vi "oa_TV Ptbypt Interpolation (NChan).vi"(5 "reset? (F)":bool, 6 "buffer size":i32[](array[numeric]), 8 "error in (no error)":errorcluster, 9 "dX":dbl[](array[numeric]), 10 "Y":cluster{dbl[]}[](array[cluster]), 11 "X":cluster{dbl[]}[](array[cluster])) -> (0 "error out":errorcluster, 1 "X0":dbl[](array[numeric]), 2 "resampled X":cluster{dbl[]}[](array[cluster]), 3 "resampled Y":cluster{dbl[]}[](array[cluster]))   [LabVIEW 2017, in "SoundVib_Torsional.lvlib"]
uses:
  <vilib>/addons/Sound and Vibration/Order Analysis/Torsional Vibration/SoundVib_Torsional.lvlib
  <vilib>/Analysis/1siggen.llb/Ramp Pattern by Samples.vi
  <vilib>/gmath/NI_Gmath.lvlib
  <vilib>/Analysis/NI_AALBase.lvlib
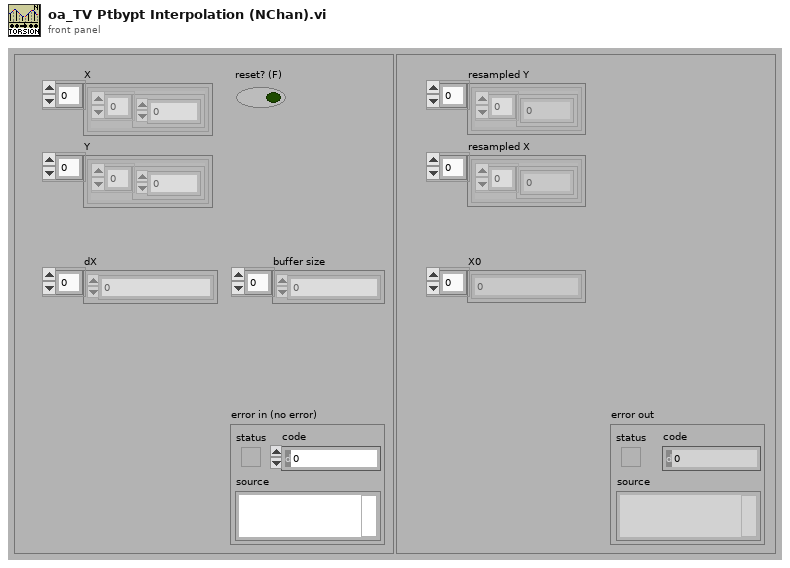
[diagram p1: front panel]
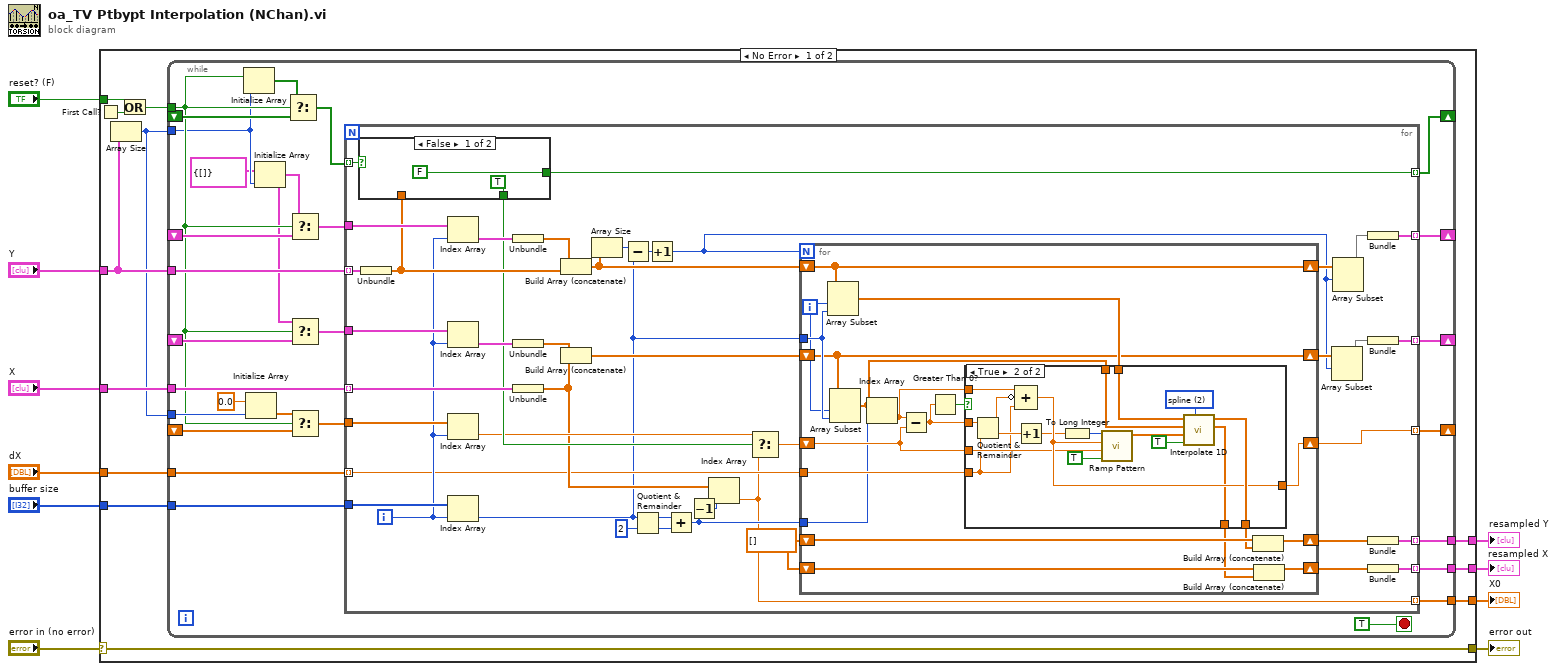
[diagram p0: block diagram]
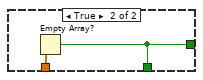
[diagram p2: hidden frame]
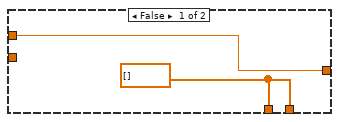
[diagram p3: hidden frame]
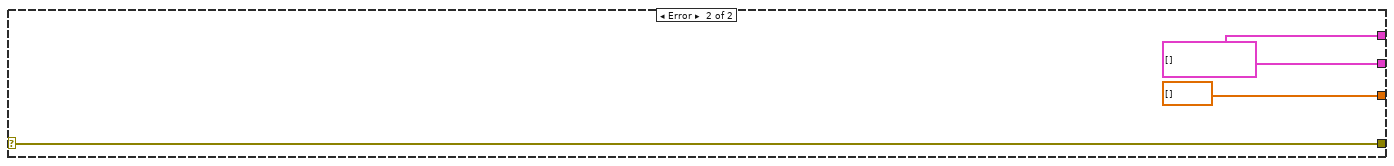
[diagram p4: hidden frame]
diagram:
  n1 = case shown="No Error" "error in (no error)" {
    selector: "error in (no error)" -> [w18 w138]
    tunnel: "buffer size" -> [w22 _]
    tunnel: "reset? (F)" -> [w20 _]
    tunnel: "X" -> [w19 _]
    tunnel: "Y" -> [w13 _]
    tunnel: [w18 w138] -> w8
    tunnel: [w15 dbl[] []] -> w4
    tunnel: [w16 w136] -> w3
    tunnel: [w14 w136] -> w2
    tunnel: "dX" -> [w11 _]
    frame No Error {
      n2 = First Call?() -> (First Call?: T/F=w21:bool)
      n3 = Array Size(array=w13) -> (size(s)=w12:i32)
      n4 = Or(x=w20, y=w21) -> (x .or. y?=w17:bool)
      n5 = while {
        tunnel: w22 -> [w44]
        tunnel: w17 -> [w28]
        tunnel: w19 -> [w45]
        tunnel: w13 -> [w47]
        shift-right: [w49] -> _
        shift-left: _ -> [w38]
        shift-right: [w46] -> _
        shift-left: _ -> [w39]
        shift-right: [w36] -> _
        shift-left: _ -> [w48]
        shift-right: [w43] -> _
        shift-left: _ -> [w33]
        tunnel: [w42] -> w16
        tunnel: [w41] -> w14
        tunnel: [w23] -> w15
        tunnel: w12 -> [w27]
        tunnel: w12 -> [w31]
        tunnel: w11 -> [w24]
        stop <- TRUE stop-if-true
        n6 = Initialize Array(w28, w27) -> (w35:bool[])
        n7 = Initialize Array(0.0 ("element"), w31) -> (w30:dbl[])
        n8 = Initialize Array(cluster{dbl[]} {[]} ("element"), w27) -> (w25:cluster{dbl[]}[])
        n9 = Select(t=w35, s=w28, f=w48) -> (s? t:f=w34:bool[])
        n10 = Select(t=w25, s=w28, f=w39) -> (s? t:f=w40:cluster{dbl[]}[])
        n11 = Select(t=w25, s=w28, f=w38) -> (s? t:f=w37:cluster{dbl[]}[])
        n12 = Select(t=w30, s=w28, f=w33) -> (s? t:f=w29:dbl[])
        n13 = for {
          tunnel: w45 -> [w93] mode=indexing
          tunnel: w44 -> [w90]
          tunnel: w47 -> [w91] mode=indexing
          tunnel: [w84] -> w42 mode=indexing
          tunnel: [w83] -> w41 mode=indexing
          tunnel: w34 -> [w76] mode=indexing
          tunnel: [w74] -> w36 mode=indexing
          tunnel: w24 -> [w65] mode=indexing
          tunnel: w40 -> [w89]
          tunnel: [w64] -> w46 mode=indexing
          tunnel: w37 -> [w92]
          tunnel: [w63] -> w49 mode=indexing
          tunnel: w29 -> [w67]
          tunnel: [w62] -> w43 mode=indexing
          tunnel: [w51] -> w23 mode=indexing
          i -> [w66]
          w85 = dbl[] []
          n14 = Unbundle(w91) -> (w75:dbl[])
          n15 = case shown="False" w76 {
            tunnel: w75 -> [_ w97]
            tunnel: [FALSE ("empty?") w96] -> w74
            tunnel: [TRUE ("empty?") w96] -> w73
            frame False {
            }
            frame True {
              n16 = Empty Array?(array=w97) -> (empty?=w96:bool)
            }
          }
          n17 = Index Array(array=w89, index=w66) -> (element=w80:cluster{dbl[]})
          n18 = Index Array(array=w92, index=w66) -> (element=w78:cluster{dbl[]})
          n19 = Index Array(array=w67, index=w66) -> (element=w72:dbl)
          n20 = Index Array(array=w90, index=w66) -> (element=w57:i32)
          n21 = Unbundle(w80) -> (w79:dbl[])
          n22 = Unbundle(w78) -> (w77:dbl[])
          n23 = Unbundle(w93) -> (w70:dbl[])
          n24 = Build Array (concatenate)(w79, w75) -> (w59:dbl[])
          n25 = Build Array (concatenate)(w77, w70) -> (w58:dbl[])
          n26 = Array Size(array=w59) -> (size(s)=w61:i32)
          n27 = Subtract(x=w61, y=w57) -> (x-y=w60:i32)
          n28 = Quotient & Remainder(x=w57, y=2) -> (x-y*floor(x/y)=w86:i32, floor(x/y)=w88:i32)
          n29 = Increment(x=w60) -> (x+1=w53:i32)
          n30 = Add(x=w86, y=w88) -> (x+y=w69:i32)
          n31 = Decrement(x=w69) -> (x-1=w68:i32)
          n32 = Index Array(array=w70, index=w68) -> (element=w51:dbl)
          n33 = Select(t=w72, s=w73, f=w51) -> (s? t:f=w71:dbl)
          n34 = for {
            N: w53 -> [_]
            shift-right: [w98] -> w56
            shift-left: w59 -> [w98]
            shift-right: [w99] -> w54
            shift-left: w58 -> [w99]
            shift-right: [w115] -> w62
            shift-left: w71 -> [w112]
            tunnel: w69 -> [w104]
            tunnel: w65 -> [w116]
            shift-right: [w108] -> w82
            shift-left: w85 -> [w114]
            shift-right: [w106] -> w81
            shift-left: w85 -> [w107]
            tunnel: w57 -> [w103]
            i -> [w102]
            n35 = Array Subset(array=w98, index=w102, length=w103) -> (w101:dbl[])
            n36 = Array Subset(array=w99, index=w102, length=w103) -> (w100:dbl[])
            n37 = Index Array(array=w100, index=w104) -> (element=w109:dbl)
            n38 = Subtract(x=w109, y=w112) -> (x-y=w111:dbl)
            n39 = Greater Than 0?(x=w111) -> (x > 0?=w110:bool)
            n40 = case shown="True" w110 {
              tunnel: w116 -> [_ w124]
              tunnel: [w118 w126] -> w115
              tunnel: [w117 w135] -> w113
              tunnel: w101 -> [_ w134]
              tunnel: w100 -> [_ w121]
              tunnel: w112 -> [w118 w125]
              tunnel: w111 -> [_ w132]
              tunnel: w109 -> [_ w129]
              tunnel: [w117 w119] -> w105
              frame False {
                w117 = dbl[] [] ("xi used")
              }
              frame True {
                w133 = 2 items=["nearest", "linear", "spline", "cubic Hermite", "Lagrange"] ("method")
                n41 = Quotient & Remainder(x=w132, y=w124) -> (x-y*floor(x/y)=w128:dbl, floor(x/y)=w130:dbl)
                n42 = Compound Arithmetic op=ADD(w129, invert w128, w124) -> (w126:dbl)
                n43 = Increment(x=w130) -> (x+1=w123:dbl)
                n44 = To Long Integer(number=w123) -> (32bit integer=w122:i32)
                n45 = call-poly <vilib>:"Ramp Pattern.vi"("exclude end?"=TRUE, "start"=w125, "end"=w126, "samples"=w122) -> ("Ramp Pattern"=w120:dbl[])  [unwired: 6 in, 1 out]
                n46 = call <vilib>:"Interpolate 1D.vi"("method"=w133, "X is monotonic"=TRUE, "xi"=w120, "X"=w121, "Y"=w134) -> ("xi used"=w119:dbl[], "yi"=w135:dbl[])  [unwired: 4 in, 1 out]
              }
            }
            n47 = Build Array (concatenate)(w114, w113) -> (w108:dbl[])
            n48 = Build Array (concatenate)(w107, w105) -> (w106:dbl[])
          }
          n49 = Array Subset(array=w54, index=w53) -> (w52:dbl[])  [unwired: 1 in]
          n50 = Array Subset(array=w56, index=w53) -> (w55:dbl[])  [unwired: 1 in]
          n51 = Bundle(w55) -> (w64:cluster{dbl[]})  [unwired: 1 in]
          n52 = Bundle(w52) -> (w63:cluster{dbl[]})  [unwired: 1 in]
          n53 = Bundle(w82) -> (w84:cluster{dbl[]})  [unwired: 1 in]
          n54 = Bundle(w81) -> (w83:cluster{dbl[]})  [unwired: 1 in]
        }
      }
    }
    frame Error {
      w136 = cluster{dbl[]}[] []
    }
  }
  "error out" <- w8
  "resampled Y" <- w3
  "resampled X" <- w2
  "X0" <- w4
